vi "Timer.vi"(8 "error in":errorcluster, 10 "target":dbl, 11 "timer status":T1) -> (0 "error out":errorcluster, 2 "time elapse":dbl, 3 "elapsed":bool)   [LabVIEW 2015]
uses:
  Controls/timer status.ctl
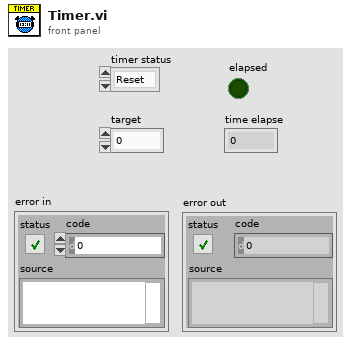
[diagram p1: front panel]
types:
  T1 = typedef "timer status.ctl" = enum16{"Reset", "Start"}
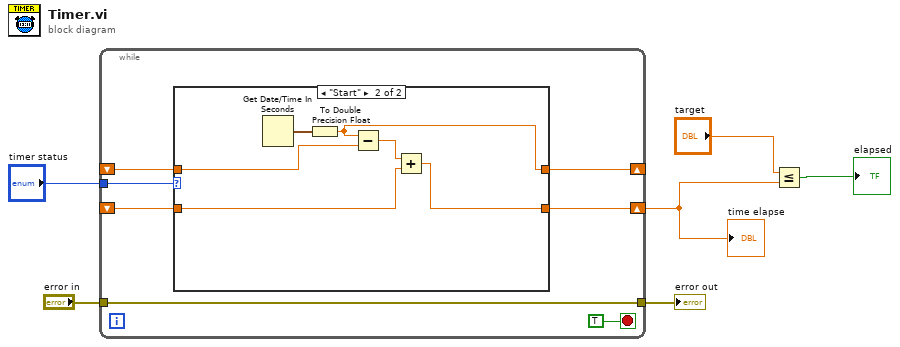
[diagram p0: block diagram]
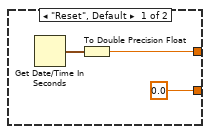
[diagram p2: hidden frame]
diagram:
  n1 = while {
    tunnel: "timer status" -> [w12]
    shift-right: [w11] -> _
    shift-left: _ -> [w9]
    shift-right: [w10] -> w5
    shift-left: _ -> [w8]
    tunnel: [w7] -> w2
    tunnel: "error in" -> [w7]
    stop <- TRUE stop-if-true
    n2 = case shown="\"Start\"" w12 {
      tunnel: [w15 w18] -> w11
      tunnel: [0.0 w19] -> w10
      tunnel: w9 -> [_ w20]
      tunnel: w8 -> [_ w17]
      frame "Reset", Default {
        n3 = Get Date/Time In Seconds() -> (seconds since 1Jan1904=w16:timestamp)
        n4 = To Double Precision Float(number=w16) -> (double precision float=w15:dbl)
      }
      frame "Start" {
        n5 = Get Date/Time In Seconds() -> (seconds since 1Jan1904=w22:timestamp)
        n6 = To Double Precision Float(number=w22) -> (double precision float=w18:dbl)
        n7 = Subtract(x=w18, y=w20) -> (x-y=w21:dbl)
        n8 = Add(x=w21, y=w17) -> (x+y=w19:dbl)
      }
    }
  }
  "time elapse" <- w5
  "error out" <- w2
  n9 = Less Or Equal?(x="target", y=w5) -> (x <= y?=→"elapsed":bool)
